vi "Test_Localization_Algorithm-2.vi"() -> ()   [LabVIEW 2020]
panel:
  out "Image":T1(plugin-control)
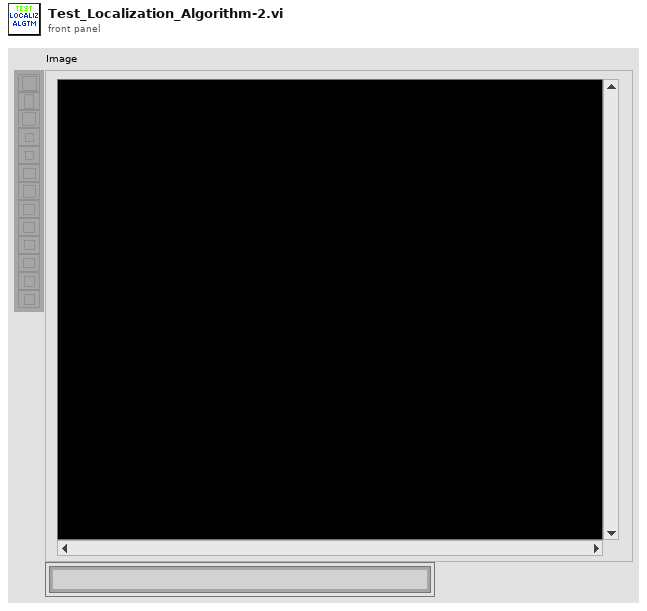
[diagram p1: front panel]
types:
  T1 = typedef "IMAQ Image.ctl" = refnum<image>
  T2 = typedef "Image Type" = u32
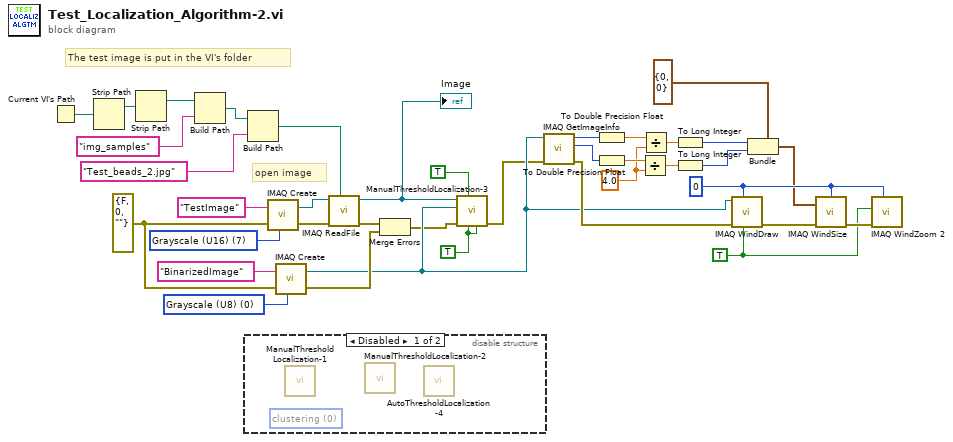
[diagram p0: block diagram]
diagram:
  w15 = 4.0 ("y")
  w14 = TRUE ("Scrollbars? (N)")
  w28 = 0 ("Window Number (0...15)")
  w8 = TRUE ("[IN] Autothreshold Images \nInstead Of Generated U8")
  w33 = T2 0 items=["Grayscale (U8)", "Grayscale (I16)", "Grayscale (SGL)", "Complex (CSG)", "RGB (U32)", "HSL (U32)", "RGB (U64)", "Grayscale (U16)"] ("Image Type")
  w37 = T2 7 items=["Grayscale (U8)", "Grayscale (I16)", "Grayscale (SGL)", "Complex (CSG)", "RGB (U32)", "HSL (U32)", "RGB (U64)", "Grayscale (U16)"] ("Image Type")
  w32 = errorcluster {"status"=FALSE, "code"=0, "source"=""} ("error in (no error)")
  # "open image"
  # "The test image is put in the VI's folder"
  n1 = Current VI's Path() -> (path=w7:path)
  n2 = Strip Path(path=w7) -> (stripped path=w6:path)  [unwired: 1 out]
  n3 = Strip Path(path=w6) -> (stripped path=w5:path)  [unwired: 1 out]
  n4 = Build Path(base path=w5, name or relative path="img_samples") -> (appended path=w3:path)
  n5 = disable-structure shown="Disabled" {
    frame Disabled {
      (unwired) 0 items=["clustering", "entropy", "metric", "moments", "inter-class variance"] ("[IN] Method")
      n6 = call "ManualThresholdLocalization-1.vi"() -> ()  [unwired: 10 in, 2 out]
      n7 = call "ManualThresholdLocalization-2.vi"() -> ()  [unwired: 10 in, 2 out]
      n8 = call "AutoThresholdLocalization-4.vi"() -> ()  [unwired: 10 in, 2 out]
    }
    frame Enabled {
    }
  }
  n9 = Build Path(base path=w3, name or relative path="Test_beads_2.jpg") -> (appended path=w1:path)
  n10 = call "IMAQ Create"("Image Name"="TestImage", "Image Type"=w37, "error in (no error)"=w32) -> ("New Image"=w35:T1, "error out"=w36:errorcluster)  [unwired: 2 in]
  n11 = call "IMAQ Create"("Image Name"="BinarizedImage", "Image Type"=w33, "error in (no error)"=w32) -> ("New Image"=w11:T1, "error out"=w30:errorcluster)  [unwired: 2 in]
  n12 = call "IMAQ ReadFile"("File Path"=w1, "error in (no error)"=w36, "Image"=w35) -> ("error out"=w31:errorcluster, "Image Out"=w13:T1)  [unwired: 4 in, 3 out]
  "Image" <- w13
  n13 = Merge Errors(w31, w30) -> (w10:errorcluster)
  n14 = call "ManualThresholdLocalization-3.vi"("[IN] Gauss Filter"=w8, "[IN] Autothreshold Images \nInstead Of Generated U8"=w8, "[IN] Median Filter"=TRUE, "error IN"=w10, "[IN] Binarized Image"=w11, "[IN] Source Image"=w13) -> ("error OUT"=w9:errorcluster)  [unwired: 4 in, 1 out]
  n15 = call "IMAQ GetImageInfo"("error in (no error)"=w9, "Image"=w11) -> ("error out"=w19:errorcluster, "Y Resolution"=w22:i32, "X Resolution"=w25:i32)  [unwired: 2 in, 5 out]
  n16 = To Double Precision Float(number=w25) -> (double precision float=w24:dbl)
  n17 = To Double Precision Float(number=w22) -> (double precision float=w21:dbl)
  n18 = Divide(x=w21, y=w15) -> (x/y=w20:dbl)
  n19 = Divide(x=w24, y=w15) -> (x/y=w23:dbl)
  n20 = To Long Integer(number=w23) -> (32bit integer=w17:i32)
  n21 = To Long Integer(number=w20) -> (32bit integer=w16:i32)
  n22 = call "IMAQ WindDraw"("Resize to Image Size? (Y)"=w14, "Window Number (0...15)"=w28, "error in (no error)"=w19, "Image"=w11) -> ("error out"=w29:errorcluster)  [unwired: 6 in, 1 out]
  n23 = Bundle(cluster=cluster{"Width":i32, "Height":i32} {"Width"=0, "Height"=0} ("Width & Height"), "Width"=w17, "Height"=w16) -> (w18:cluster{"Width":i32, "Height":i32})
  n24 = call "IMAQ WindSize"("error in (no error)"=w29, "Width & Height"=w18, "Window Number"=w28) -> ("error out"=w27:errorcluster)  [unwired: 3 in, 2 out]
  n25 = call "IMAQ WindZoom 2"("Window Number (0...15)"=w28, "error in (no error)"=w27, "Zoom to Fit? (False)"=w14) -> ()  [unwired: 5 in, 4 out]
